vi "DispenseCycle.vi"(5 "DispenseAnalyte":string, 6 "LastWasteAnalyte":string, 7 "pullAnalyte":string, 8 "PullPush":bool=TRUE, 9 "speed_uL_s":dbl, 10 "volume_uL":dbl, 11 "Pump_Refnum":refnum<k24>) -> (3 "Pump":refnum<k24>)   [LabVIEW 2020]
uses:
  D:/PumpAutomation2/DEMPBot2/PumpAdapter.exe
  PumpAdapter.exe
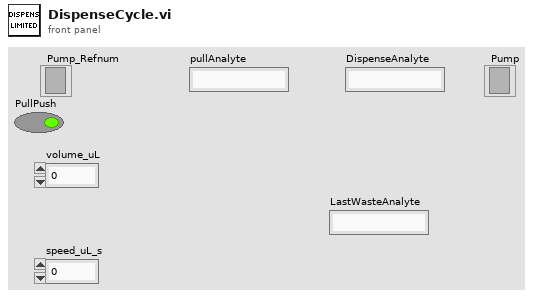
[diagram p1: front panel]
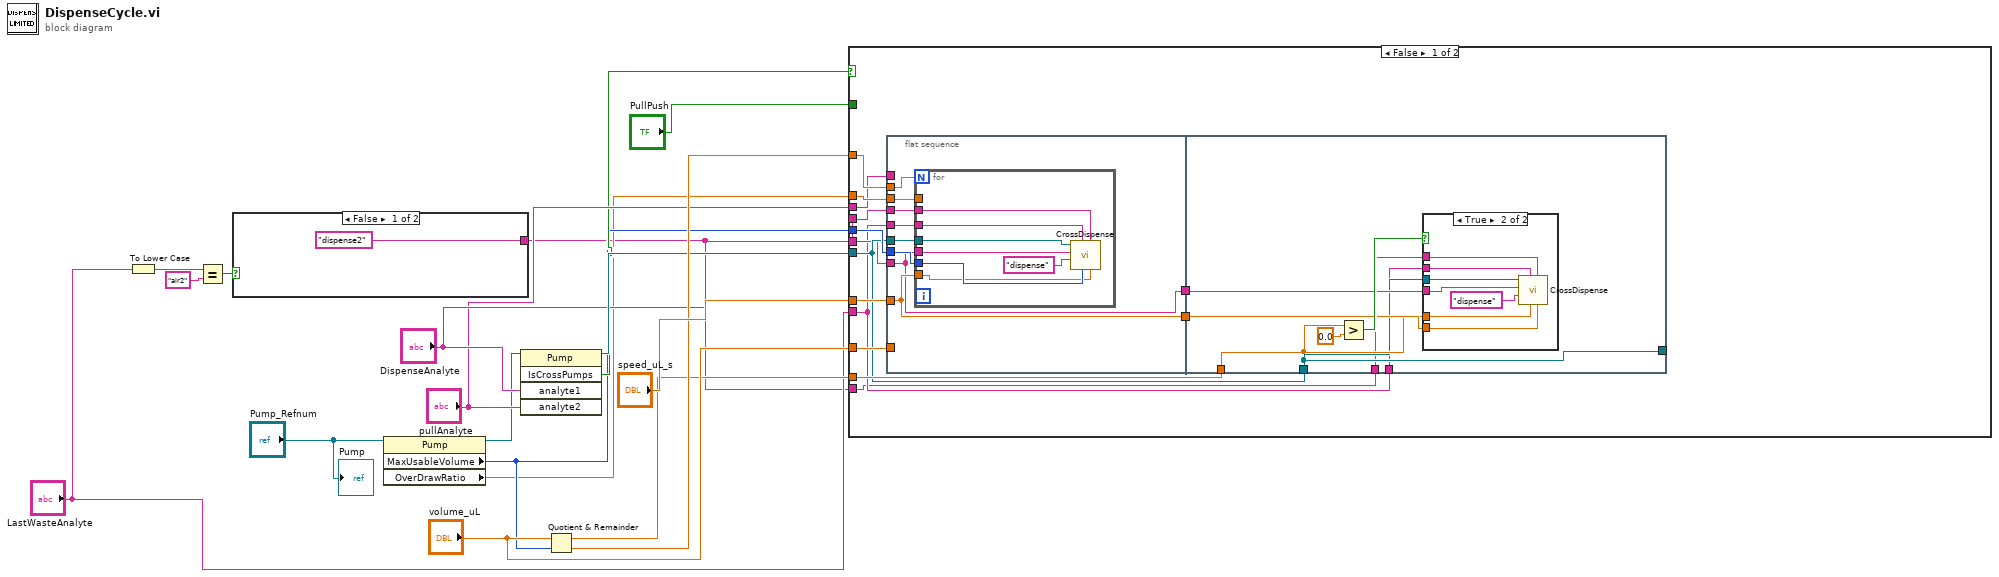
[diagram p0: block diagram]
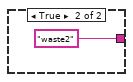
[diagram p2: hidden frame]
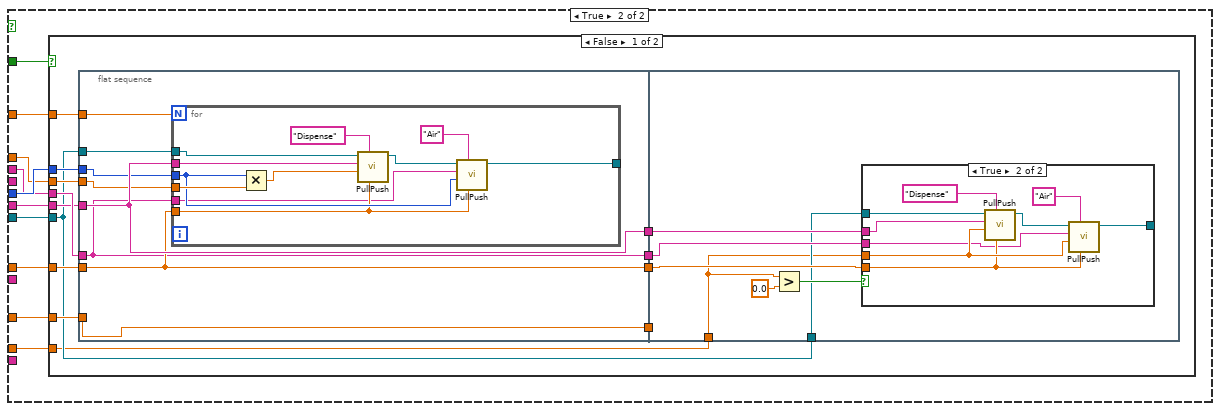
[diagram p4: hidden frame]
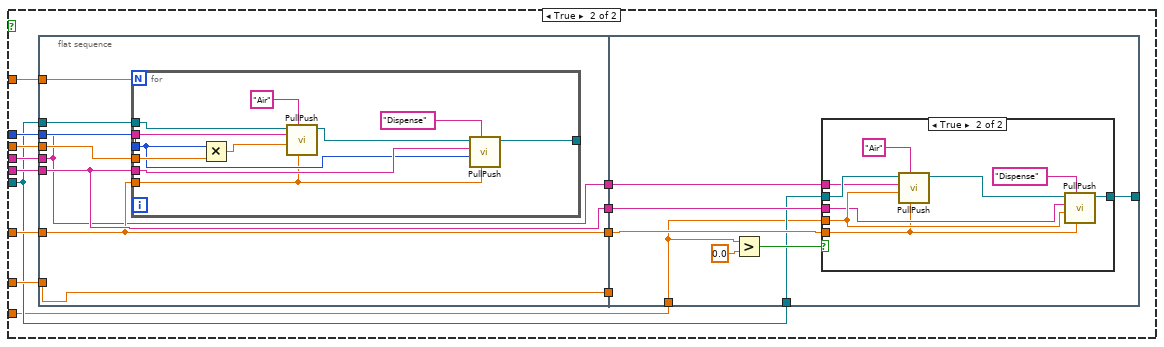
[diagram p6: hidden frame]
diagram:
  n1 = To Lower Case(string="LastWasteAnalyte") -> (all lower case string=w4:string)
  n2 = Equal?(x=w4, y="air2" ("wasteOutletAnalyte")) -> (x = y?=w2:bool)
  n3 = case shown="False" w2 {
    tunnel: ["dispense2" "waste2" ("wasteLine")] -> w1
    frame False {
    }
    frame True {
    }
  }
  n4 = property class="Pump"(reference="Pump_Refnum") -> (reference out=w9:refnum<k24>, "MaxUsableVolume"=w8:i32, "OverDrawRatio"=w7:dbl)  [unwired: 1 in, 1 out]
  n5 = invoke class="Pump" method="IsCrossPumps"(reference=w9, "analyte1"="DispenseAnalyte", "analyte2"="pullAnalyte") -> (reference out=w13:refnum<k24>, "IsCrossPumps"=w10:bool)  [unwired: 2 in, 3 out]
  n6 = Quotient & Remainder(x="volume_uL", y=w8) -> (x-y*floor(x/y)=w15:dbl, floor(x/y)=w16:dbl)
  n7 = case shown="False" w10 {
    tunnel: "volume_uL" -> [w31 w74]
    tunnel: "speed_uL_s" -> [w32 w73]
    tunnel: w8 -> [w33 w72]
    tunnel: w7 -> [w29 w71]
    tunnel: w16 -> [w34 w70]
    tunnel: w15 -> [w30 w69]
    tunnel: "PullPush" -> [_ w68]
    tunnel: w13 -> [w26 w65]
    tunnel: "DispenseAnalyte" -> [w24 w67]
    tunnel: "pullAnalyte" -> [w25 w66]
    tunnel: "LastWasteAnalyte" -> [w23 _]
    tunnel: w1 -> [w22 _]
    tunnel: w1 -> [w21 _]
    frame False {
      n8 = flat-sequence {
        tunnel: w24 -> [w37]
        tunnel: w32 -> [w40]
        tunnel: w25 -> [_]
        tunnel: w31 -> [_]
        tunnel: [w40] -> w28
        tunnel: [w37] -> w27
        tunnel: w34 -> [w42]
        tunnel: w26 -> [w41]
        tunnel: w33 -> [w39]
        tunnel: w29 -> [w38]
        tunnel: w23 -> [w36]
        tunnel: w22 -> [w35]
        tunnel: w28 -> [w55]
        tunnel: w27 -> [w54]
        tunnel: w26 -> [w52]
        tunnel: w30 -> [w53]
        tunnel: [w52] -> _
        tunnel: w23 -> [w51]
        tunnel: w21 -> [w50]
        frame #0 {
          n9 = for {
            N: w42 -> [_]
            tunnel: w41 -> [w49]
            tunnel: w40 -> [w47]
            tunnel: w39 -> [w48]
            tunnel: w38 -> [_]
            tunnel: w37 -> [w45]
            tunnel: w36 -> [w44]
            tunnel: w35 -> [w43]
            n10 = call "CrossDispense.vi"("speed_uL_s"=w47, "wasteLine"=w43, "drawVolume_ul"=w48, "airWaste2"=w44, "dispenseLine"="dispense", "drawAnalyte"=w45, "Pump in"=w49) -> ()  [unwired: 3 in, 2 out]
          }
        }
        frame #1 {
          n11 = Greater?(x=w53, y=0.0) -> (0:w57:bool)
          n12 = case shown="True" w57 {
            tunnel: w53 -> [_ w62]
            tunnel: w52 -> [_ w64]
            tunnel: w55 -> [_ w61]
            tunnel: w54 -> [_ w63]
            tunnel: w51 -> [_ w59]
            tunnel: w50 -> [_ w58]
            frame False {
            }
            frame True {
              n13 = call "CrossDispense.vi"("speed_uL_s"=w61, "wasteLine"=w58, "drawVolume_ul"=w62, "airWaste2"=w59, "dispenseLine"="dispense", "drawAnalyte"=w63, "Pump in"=w64) -> ()  [unwired: 3 in, 2 out]
            }
          }
        }
      }
    }
    frame True {
      n14 = case shown="False" w68 {
        tunnel: w74 -> [w77 w132]
        tunnel: w66 -> [w83 w131]
        tunnel: w73 -> [w78 w130]
        tunnel: w67 -> [w79 w129]
        tunnel: w72 -> [w82 w128]
        tunnel: w71 -> [w81 w127]
        tunnel: w65 -> [w76 w126]
        tunnel: w70 -> [w80 w125]
        tunnel: w69 -> [w75 w124]
        frame False {
          n15 = flat-sequence {
            tunnel: w79 -> [w92]
            tunnel: w78 -> [w91]
            tunnel: w83 -> [w88]
            tunnel: w77 -> [w95]
            tunnel: [w95] -> w87
            tunnel: [w88] -> w86
            tunnel: [w91] -> w85
            tunnel: [w92] -> w84
            tunnel: w80 -> [w94]
            tunnel: w76 -> [w93]
            tunnel: w82 -> [w90]
            tunnel: w81 -> [w89]
            tunnel: w87 -> [_]
            tunnel: w86 -> [w111]
            tunnel: w85 -> [w110]
            tunnel: w84 -> [w109]
            tunnel: w76 -> [w108]
            tunnel: w75 -> [w107]
            frame #0 {
              n16 = for {
                N: w94 -> [_]
                tunnel: w93 -> [w106]
                tunnel: w92 -> [w99]
                tunnel: w91 -> [w100]
                tunnel: w90 -> [w101]
                tunnel: w89 -> [w105]
                tunnel: w88 -> [w98]
                tunnel: [w102] -> _
                n17 = Multiply(x=w101, y=w105) -> (x*y=w104:dbl)
                n18 = call "PullPush.vi"("speed_uL_s"=w100, "pushTo"="Dispense", "volume_uL"=w104, "pullFrom"=w99, ".NET Refnum in"=w106) -> (".NET Refnum out"=w103:refnum<k24>)  [unwired: 6 in]
                n19 = call "PullPush.vi"("speed_uL_s"=w100, "pushTo"="Air" ("analyte"), "volume_uL"=w101, "pullFrom"=w98, ".NET Refnum in"=w103) -> (".NET Refnum out"=w102:refnum<k24>)  [unwired: 6 in]
              }
            }
            frame #1 {
              n20 = Greater?(x=w107, y=0.0) -> (0:w113:bool)
              n21 = case shown="True" w113 {
                tunnel: w107 -> [_ w120]
                tunnel: [w114 w121] -> _
                tunnel: w108 -> [w114 w123]
                tunnel: w111 -> [_ w116]
                tunnel: w110 -> [_ w119]
                tunnel: w109 -> [_ w115]
                frame False {
                }
                frame True {
                  n22 = call "PullPush.vi"("speed_uL_s"=w119, "pushTo"="Dispense", "volume_uL"=w120, "pullFrom"=w115, ".NET Refnum in"=w123) -> (".NET Refnum out"=w122:refnum<k24>)  [unwired: 6 in]
                  n23 = call "PullPush.vi"("speed_uL_s"=w119, "pushTo"="Air" ("analyte"), "volume_uL"=w120, "pullFrom"=w116, ".NET Refnum in"=w122) -> (".NET Refnum out"=w121:refnum<k24>)  [unwired: 6 in]
                }
              }
            }
          }
        }
        frame True {
          n24 = flat-sequence {
            tunnel: w129 -> [w141]
            tunnel: w130 -> [w140]
            tunnel: w131 -> [w137]
            tunnel: w132 -> [w144]
            tunnel: [w144] -> w136
            tunnel: [w137] -> w135
            tunnel: [w140] -> w134
            tunnel: [w141] -> w133
            tunnel: w125 -> [w143]
            tunnel: w126 -> [w142]
            tunnel: w128 -> [w139]
            tunnel: w127 -> [w138]
            tunnel: w136 -> [_]
            tunnel: w135 -> [w161]
            tunnel: w134 -> [w160]
            tunnel: w133 -> [w159]
            tunnel: w126 -> [w158]
            tunnel: w124 -> [w157]
            tunnel: [w156] -> _
            frame #0 {
              n25 = for {
                N: w143 -> [_]
                tunnel: w142 -> [w155]
                tunnel: w141 -> [w149]
                tunnel: w140 -> [w146]
                tunnel: w139 -> [w147]
                tunnel: w138 -> [w154]
                tunnel: w137 -> [w153]
                tunnel: [w148] -> _
                n26 = Multiply(x=w147, y=w154) -> (x*y=w152:dbl)
                n27 = call "PullPush.vi"("speed_uL_s"=w146, "pushTo"="Air" ("analyte"), "volume_uL"=w152, "pullFrom"=w153, ".NET Refnum in"=w155) -> (".NET Refnum out"=w150:refnum<k24>)  [unwired: 6 in]
                n28 = call "PullPush.vi"("speed_uL_s"=w146, "pushTo"="Dispense", "volume_uL"=w147, "pullFrom"=w149, ".NET Refnum in"=w150) -> (".NET Refnum out"=w148:refnum<k24>)  [unwired: 6 in]
              }
            }
            frame #1 {
              n29 = Greater?(x=w157, y=0.0) -> (0:w163:bool)
              n30 = case shown="True" w163 {
                tunnel: w157 -> [_ w169]
                tunnel: [w164 w171] -> w156
                tunnel: w158 -> [w164 w173]
                tunnel: w161 -> [_ w168]
                tunnel: w160 -> [_ w166]
                tunnel: w159 -> [_ w167]
                frame False {
                }
                frame True {
                  n31 = call "PullPush.vi"("speed_uL_s"=w166, "pushTo"="Air" ("analyte"), "volume_uL"=w169, "pullFrom"=w168, ".NET Refnum in"=w173) -> (".NET Refnum out"=w172:refnum<k24>)  [unwired: 6 in]
                  n32 = call "PullPush.vi"("speed_uL_s"=w166, "pushTo"="Dispense", "volume_uL"=w169, "pullFrom"=w167, ".NET Refnum in"=w172) -> (".NET Refnum out"=w171:refnum<k24>)  [unwired: 6 in]
                }
              }
            }
          }
        }
      }
    }
  }
  "Pump" <- "Pump_Refnum"
